vi "applicationSettings.vi"() -> ()   [LabVIEW 2018]
panel:
  in  "Address":string
  in  "Use Address":bool
  in  "Dev Mode":bool
  # "Settings"
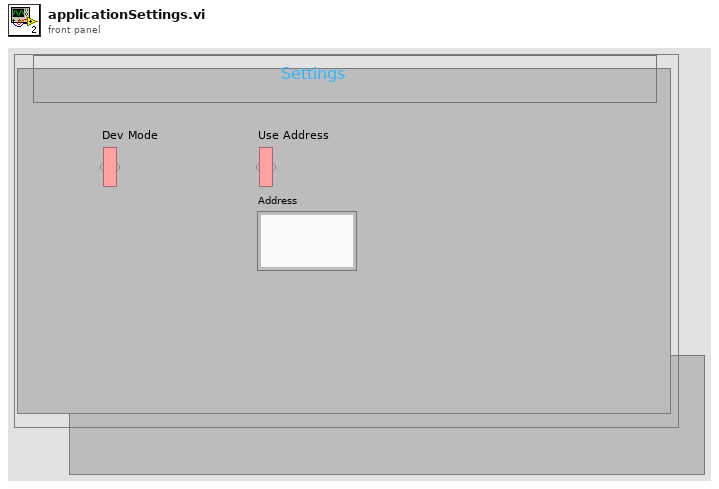
[diagram p1: front panel]
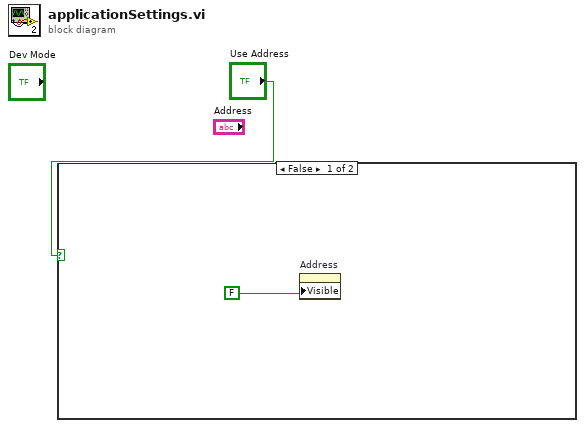
[diagram p0: block diagram]
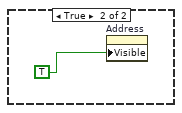
[diagram p2: hidden frame]
diagram:
  n1 = case shown="False" "Use Address" {
    frame False {
      n2 = property on="Address" class="Str"("Visible"=FALSE) -> ()  [unwired: 2 in, 2 out]
    }
    frame True {
      n3 = property on="Address" class="Str"("Visible"=TRUE) -> ()  [unwired: 2 in, 2 out]
    }
  }
